vi "Relative to absolute path.vi"(1 "Relative Path":path) -> (0 "Absolute Path":path)   [LabVIEW 2020]
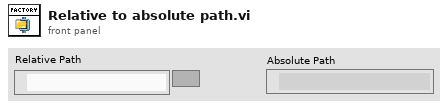
[diagram p1: front panel]
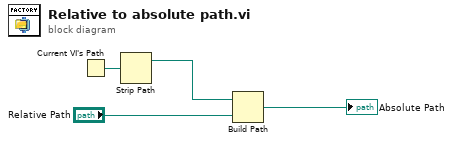
[diagram p0: block diagram]
diagram:
  n1 = Current VI's Path() -> (path=w4:path)
  n2 = Strip Path(path=w4) -> (stripped path=w3:path)  [unwired: 1 out]
  n3 = Build Path(base path=w3, name or relative path="Relative Path") -> (appended path=→"Absolute Path":path)
